vi "Initialize.vi"(4 "verify server (true)":bool=TRUE, 6 "Version (no version)":string, 7 "API Root":string, 8 "error in (no error)":errorcluster, 9 "Port (protocol specific)":u16, 10 "Base URL":string, 11 "ByteGSAPIBase in":refnum<class "ByteRESTBase.lvclass">) -> (0 "error out":errorcluster, 3 "ByteGSAPIBase out":refnum<class "ByteRESTBase.lvclass">)   [LabVIEW 2019, in "ByteREST.lvlib" / "ByteRESTBase.lvclass"]
doc: "Apre una nuova connessione HTTP e setta il content type a \"application/json\""
uses:
  ByteRESTBase.lvclass
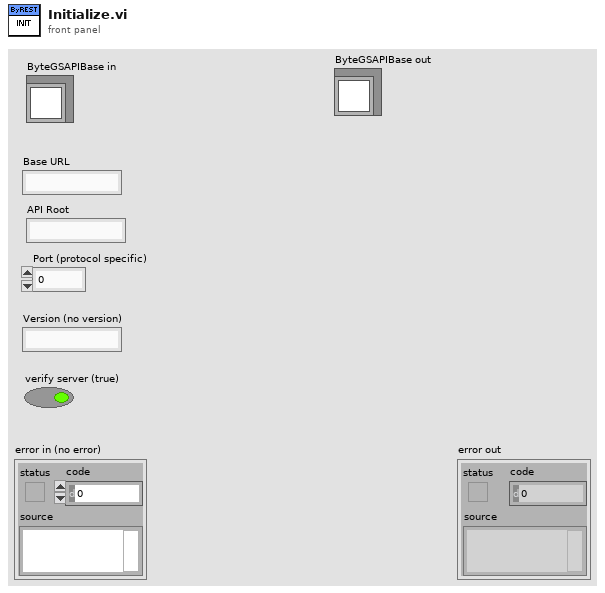
[diagram p1: front panel]
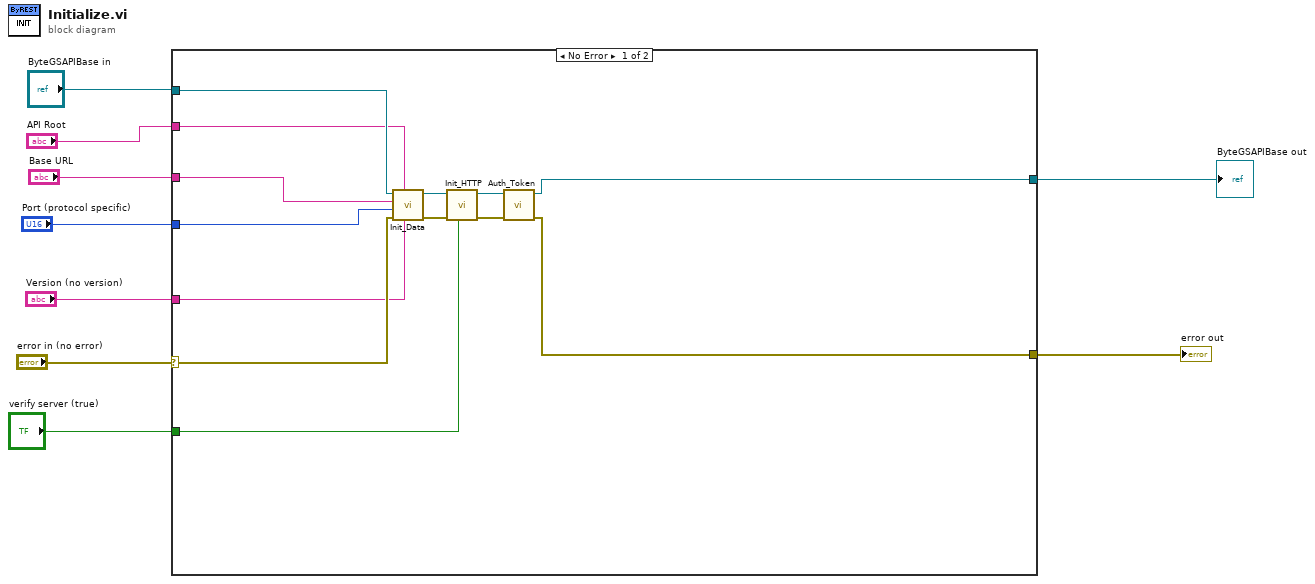
[diagram p0: block diagram]
diagram:
  n1 = case shown="No Error" "error in (no error)" {
    selector: "error in (no error)" -> [w16 w24]
    tunnel: [w11 w24] -> w8
    tunnel: [w12 w23] -> w5
    tunnel: "ByteGSAPIBase in" -> [w20 w23]
    tunnel: "Base URL" -> [w18 _]
    tunnel: "Port (protocol specific)" -> [w17 _]
    tunnel: "Version (no version)" -> [w15 _]
    tunnel: "API Root" -> [w19 _]
    tunnel: "verify server (true)" -> [w10 _]
    frame No Error {
      n2 = call "Init_Data.vi"("Version (no version)"=w15, "API Root"=w19, "error in (no error)"=w16, "Port (protocol specific)"=w17, "Base URL"=w18, "ByteGSAPIBase in"=w20) -> ("error out"=w21:errorcluster, "ByteGSAPIBase out"=w22:refnum<class "ByteRESTBase.lvclass">)  [unwired: 4 in]
      n3 = call "Init_HTTP.vi"("verify server(true)"=w10, "error in (no error)"=w21, "ByteRESTBase in"=w22) -> ("error out"=w13:errorcluster, "ByteRESTBase out"=w14:refnum<class "ByteRESTBase.lvclass">)  [unwired: 7 in]
      n4 = call "Auth_Token.vi"("error in (no error)"=w13, "ByteGSAPIBase in"=w14) -> ("error out"=w11:errorcluster, "ByteGSAPIBase out"=w12:refnum<class "ByteRESTBase.lvclass">)  [unwired: 8 in]
    }
    frame Error {
    }
  }
  "error out" <- w8
  "ByteGSAPIBase out" <- w5
